vi "add new mapping by data type.vi"(8 "data type":T2, 9 "sink name":string, 10 "source name":string, 11 "mappings":T1[](array[typedef])) -> (3 "mappings out":T1[](array[typedef]))   [LabVIEW 2014, in "base TBM sequencer configuration.lvclass"]
uses:
  base TBM sequencer configuration.lvclass
  <vilib>/NI/Tag Bus/table/mapping specification.ctl
  <vilib>/NI/Tag Bus/tag/Data Type.ctl
  <vilib>/NI/Tag Bus/table/mapping.ctl
  <vilib>/NI/Tag Bus/table/data table.lvlib
  <vilib>/NI/Tag Bus/tag/tag descriptor.lvclass
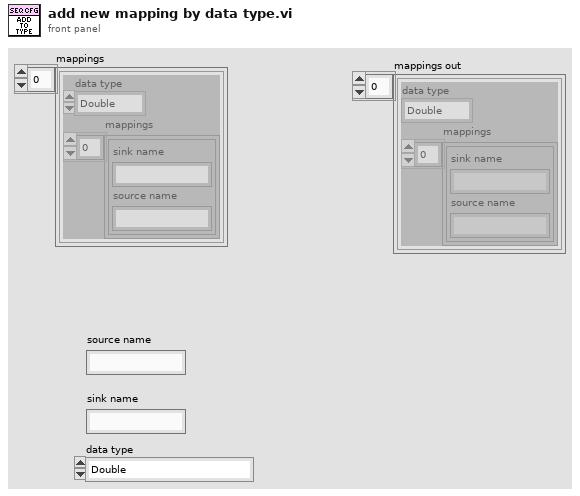
[diagram p1: front panel]
types:
  T1 = typedef "tag bus.lvlib/data table.lvlib/mapping specification.ctl" = cluster{"data type":T2, "mappings":T3[]}
  T2 = typedef "tag bus.lvlib/tag descriptor.lvclass/Data Type.ctl" = enum16{"Double", "Single", "I64", "I32", "I16", "I8", "U64", "U32", "U16", "U8", "Boolean", "String", "Array of Double", "Array of Single", "Array of I64", "Array of I32", "Array of I16", "Array of I8", "Array of U64", "Array of U32", "Array of U16", "Array of U8", "Array of Boolean", "Array of String"}
  T3 = typedef "tag bus.lvlib/data table.lvlib/mapping.ctl" = cluster{"sink name":string, "source name":string}
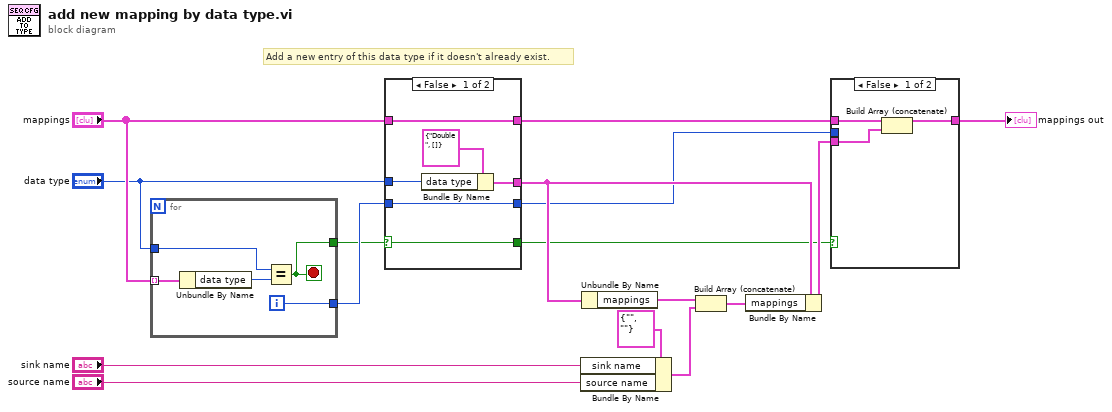
[diagram p0: block diagram]
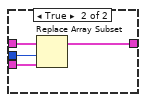
[diagram p2: hidden frame]
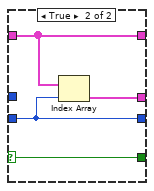
[diagram p3: hidden frame]
diagram:
  # "Add a new entry of this data type if it doesn't already exist."
  n1 = for {
    tunnel: "mappings" -> [w17] mode=indexing
    tunnel: "data type" -> [w20]
    tunnel: [w19] -> w9
    tunnel: [w18] -> w8
    i -> [w19]
    stop <- w18 stop-if-true
    n2 = Unbundle By Name(w17) -> ("data type"=w21:T2)
    n3 = Equal?(x=w20, y=w21) -> (x = y?=w18:bool)
  }
  n4 = case shown="False" w8 {
    selector: w8 -> [w23 w29]
    tunnel: "mappings" -> [w24 w30]
    tunnel: w9 -> [w22 w28]
    tunnel: [w25 w31] -> w14
    tunnel: [w24 w30] -> w13
    tunnel: "data type" -> [w26 _]
    tunnel: [w23 w29] -> w1
    tunnel: [w22 w28] -> w2
    frame False {
      n5 = Bundle By Name(cluster=T1 {"data type"=enum."Double", "mappings"=[]} ("element"), "data type"=w26) -> (w25:T1)
    }
    frame True {
      n6 = Index Array(array=w30, index=w28) -> (element=w31:T1)
    }
  }
  n7 = Bundle By Name(cluster=T3 {"sink name"="", "source name"=""} ("mapping"), "sink name"="sink name", "source name"="source name") -> (w12:T3)
  n8 = Unbundle By Name(w14) -> ("mappings"=w10:T3[])
  n9 = Build Array (concatenate)(w10, w12) -> (w15:T3[])
  n10 = Bundle By Name(cluster=w14, "mappings"=w15) -> (w16:T1)
  n11 = case shown="False" w1 {
    tunnel: w16 -> [w33 w38]
    tunnel: w13 -> [w34 w37]
    tunnel: [w32 w36] -> w3
    tunnel: w2 -> [_ w35]
    frame False {
      n12 = Build Array (concatenate)(w34, w33) -> (w32:T1[])
    }
    frame True {
      n13 = Replace Array Subset(array=w37, new element=w38, index=w35) -> (w36:T1[])
    }
  }
  "mappings out" <- w3
